vi "Initialize.vi"(8 "error in (no error)":errorcluster, 9 "Variable Names":string[](array[string]), 10 "Description":string, 11 "Pipe Name":string) -> (0 "error out":errorcluster, 3 "Pipe":T1)   [LabVIEW 2022 SP3, in "Pipes.lvlib"]
uses:
  Pipes.lvlib
  Controls/Pipe.ctl
  Controls/Pipe Definition.ctl
  Controls/Token Type.ctl
  Controls/Token.ctl
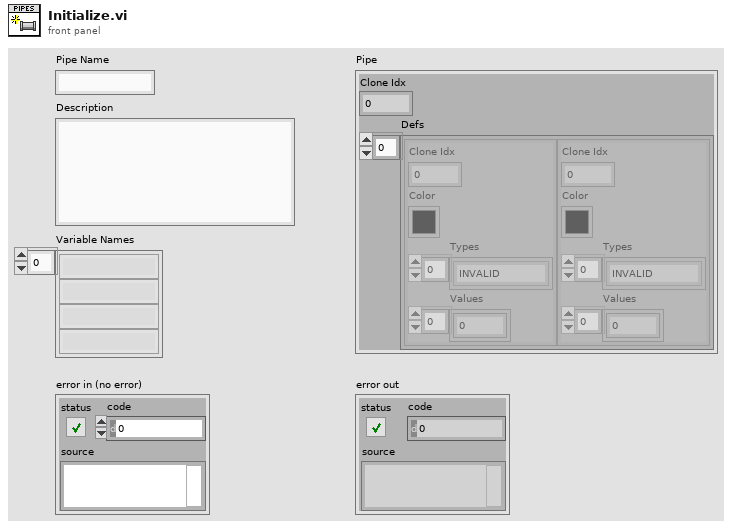
[diagram p1: front panel]
types:
  T1 = typedef "Pipes.lvlib/Pipe.ctl" = cluster{"Clone Idx":i32, "Defs":T2[]}
  T2 = typedef "Pipes.lvlib/Pipe Definition.ctl" = cluster{"Clone Idx":i32, "Color":u32, "Types":T3[], "Values":dbl[]}
  T3 = typedef "Pipes.lvlib/Token Type.ctl" = enum8{"INVALID", "NOT", "AND", "OR", "EE", "NE", "LT", "GT", "LTE", "GTE", "PLUS", "MINUS", "MULTIPLY", "DIVIDE", "MODULUS", "LPAREN", "RPAREN", "LITERAL", "IDENTIFIER", "DEFINITION"}
  T4 = typedef "Pipes.lvlib/Token.ctl" = cluster{"Offset":i32, "Type":T3, "Value":string}
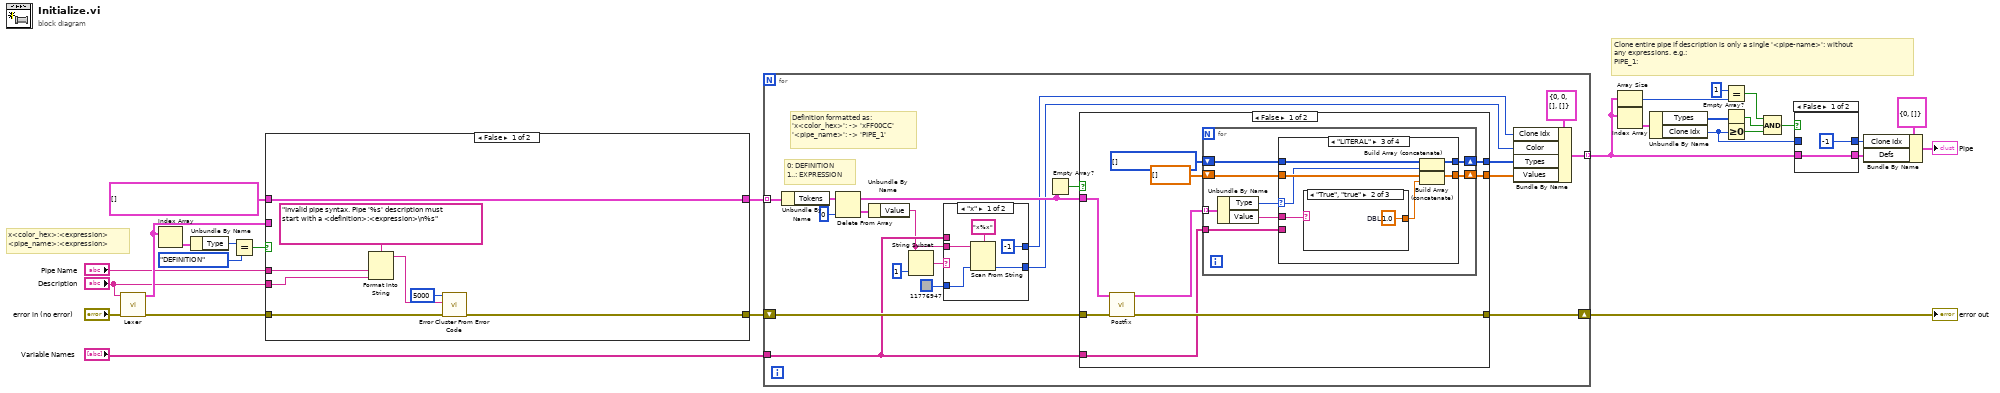
[diagram p0: block diagram]
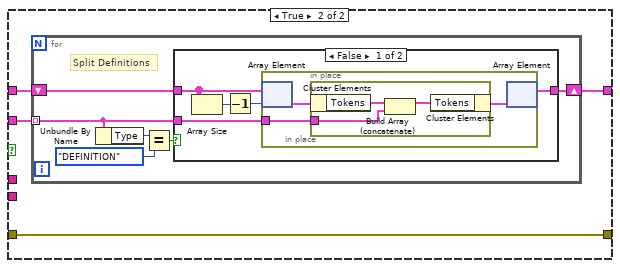
[diagram p3: hidden frame]
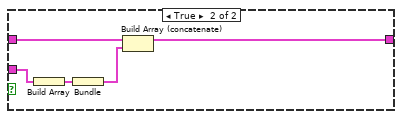
[diagram p4: hidden frame]
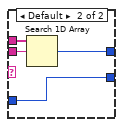
[diagram p5: hidden frame]
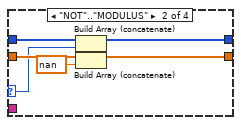
[diagram p7: hidden frame]
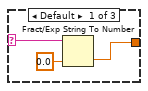
[diagram p8: hidden frame]
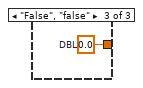
[diagram p9: hidden frame]
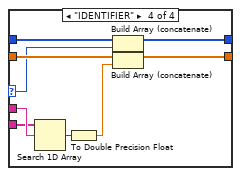
[diagram p10: hidden frame]
diagram:
  # "Clone entire pipe if description is only a single '<pipe-name>': without\nany expressions. e.g.:\nPIPE_1:"
  # "x<color_hex>:<expression>\n<pipe_name>:<expression>"
  n1 = call "Lexer.vi"("error in (no error)"="error in (no error)", "Input"="Description") -> ("error out"=w15:errorcluster, "Tokens"=w21:T4[])  [unwired: 8 in]
  n2 = Index Array(array=w21) -> (element=w18:T4)  [unwired: 1 in]
  n3 = Unbundle By Name(w18) -> ("Type"=w19:T3)
  n4 = Equal?(x=w19, y=Token_Type."DEFINITION" ("x")) -> (x = y?=w17:bool)
  n5 = case shown="False" w17 {
    tunnel: cluster{"Tokens":T4[]}[] [] ("Defs") -> [w35 w40]
    tunnel: [w35 w39] -> w23
    tunnel: w21 -> [_ w38]
    tunnel: [w34 w37] -> w16
    tunnel: w15 -> [w36 w37]
    tunnel: "Description" -> [w30 _]
    tunnel: "Pipe Name" -> [w32 _]
    frame False {
      n6 = Format Into String(format string="Invalid pipe syntax. Pipe '%s' description must start with a <definition>:<expression>\n%s" ("error message (\"\")"), w32, w30) -> (resulting string=w29:string)  [unwired: 2 in, 1 out]
      n7 = call <vilib>:"Error Cluster From Error Code.vi"("error in (no error)"=w36, "error message (\"\")"=w29, "error code (0)"=5000) -> ("error out"=w34:errorcluster)  [unwired: 6 in]
    }
    frame True {
      n8 = for {
        tunnel: w38 -> [w43] mode=indexing
        shift-right: [w42] -> w39
        shift-left: w40 -> [w44]
        # "Split Definitions"
        n9 = Unbundle By Name(w43) -> ("Type"=w46:T3)
        n10 = Equal?(x=w46, y=Token_Type."DEFINITION" ("x")) -> (x = y?=w41:bool)
        n11 = case shown="False" w41 {
          tunnel: w44 -> [w51 w62]
          tunnel: w43 -> [w48 w61]
          tunnel: [w47 w58] -> w42
          frame False {
            n12 = Array Size(array=w51) -> (size(s)=w50:i32)
            n13 = Decrement(x=w50) -> (x-1=w49:i32)
            n14 = in-place {
              in-place-border: w48 -> [w53]
              n15 = in-place-array #1(w51, w49) -> (w54:cluster{"Tokens":T4[]})
              n16 = in-place {
                in-place-border: w53 -> [w55]
                n17 = in-place-cluster #2(w54) -> ("Tokens"=w57:T4[])
                n18 = Build Array (concatenate)(w57, w55) -> (w56:T4[])
                n19 = in-place-cluster #2("Tokens"=w56) -> (w52:cluster{"Tokens":T4[]})
              }
              n20 = in-place-array #1(w52) -> (w47:cluster{"Tokens":T4[]}[])  [unwired: 1 out]
            }
          }
          frame True {
            n21 = Build Array(w61) -> (w60:T4[])
            n22 = Bundle(w60) -> (w59:cluster{T4[]})  [unwired: 1 in]
            n23 = Build Array (concatenate)(w62, w59) -> (w58:cluster{"Tokens":T4[]}[])
          }
        }
      }
    }
  }
  n24 = for {
    shift-right: [w80] -> w25
    shift-left: w16 -> [w81]
    tunnel: w23 -> [w78] mode=indexing
    tunnel: "Variable Names" -> [w69]
    tunnel: [w70] -> w5 mode=indexing
    # "Definition formatted as:\n'x<color_hex>': -> 'xFF00CC'\n'<pipe_name>': -> 'PIPE_1'"
    # "0: DEFINITION\n1..: EXPRESSION"
    n25 = Unbundle By Name(w78) -> ("Tokens"=w77:T4[])
    n26 = Delete From Array(array=w77, index=0) -> (deleted portion=w75:T4, array with subset deleted=w72:T4[])  [unwired: 1 in]
    n27 = Unbundle By Name(w75) -> ("Value"=w68:string)
    n28 = String Subset(string=w68, length (rest)=1 ("length (rest)")) -> (substring=w66:string)  [unwired: 1 in]
    n29 = case shown="\"x\"" w66 {
      tunnel: w69 -> [_ w90]
      tunnel: w68 -> [w86 w89]
      tunnel: [-1 ("index of element") w88] -> w65
      tunnel: [w84 w87] -> w64
      tunnel: u32 11776947 ("Color") -> [w85 w87]
      frame "x" {
        n30 = Scan From String(format string="x%x", input string=w86, default 1=w85) -> (output 1=w84:u32)  [unwired: 2 in, 3 out]
      }
      frame Default {
        n31 = Search 1D Array(1D array=w90, element=w89) -> (index of element=w88:i32)  [unwired: 1 in]
      }
    }
    n32 = Empty Array?(array=w72) -> (empty?=w71:bool)
    n33 = case shown="False" w71 {
      tunnel: w81 -> [w99 w137]
      tunnel: [w98 w137] -> w80
      tunnel: [w95 _] -> w74
      tunnel: [w93 _] -> w73
      tunnel: w69 -> [w92 _]
      tunnel: w72 -> [w91 _]
      frame False {
        w96 = T3[] [] items=["INVALID", "NOT", "AND", "OR", "EE", "NE", "LT", "GT", "LTE", "GTE", "PLUS", "MINUS", "MULTIPLY", "DIVIDE", "MODULUS", "LPAREN", "RPAREN", "LITERAL", "IDENTIFIER", "DEFINITION"]
        n34 = call "Postfix.vi"("error in (no error)"=w99, "Tokens"=w91) -> ("error out"=w98:errorcluster, "Postfix"=w97:T4[])  [unwired: 8 in]
        n35 = for {
          tunnel: w97 -> [w107] mode=indexing
          shift-right: [w105] -> w95
          shift-left: w96 -> [w104]
          shift-right: [w102] -> w93
          shift-left: dbl[] [] ("Values") -> [w103]
          tunnel: w92 -> [w100]
          n36 = Unbundle By Name(w107) -> ("Type"=w106:T3, "Value"=w101:string)
          n37 = case shown="\"LITERAL\"" w106 {
            selector: w106 -> [_ w111 w118 w132]
            tunnel: [w109 w113 w120 w134] -> w105
            tunnel: w104 -> [w109 w115 w122 w136]
            tunnel: w103 -> [w108 w114 w121 w135]
            tunnel: [w108 w112 w119 w133] -> w102
            tunnel: w101 -> [_ _ w117 w131]
            tunnel: w100 -> [_ _ _ w130]
            frame "INVALID", "LPAREN", "RPAREN", "DEFINITION" {
            }
            frame "NOT".."MODULUS" {
              n38 = Build Array (concatenate)(w115, w111) -> (w113:T3[])
              n39 = Build Array (concatenate)(w114, nan) -> (w112:dbl[])
            }
            frame "LITERAL" {
              n40 = case shown="\"True\", \"true\"" w117 {
                selector: w117 -> [w125 _ _]
                tunnel: [w123 w126 w127] -> w116
                frame Default {
                  n41 = Fract/Exp String To Number(string=w125, default (0 dbl)=0.0 ("DBL")) -> (number=w123:dbl)  [unwired: 2 in, 1 out]
                }
                frame "True", "true" {
                  w126 = 1.0  # DBL
                }
                frame "False", "false" {
                  w127 = 0.0  # DBL
                }
              }
              n42 = Build Array (concatenate)(w122, w118) -> (w120:T3[])
              n43 = Build Array (concatenate)(w121, w116) -> (w119:dbl[])
            }
            frame "IDENTIFIER" {
              n44 = Search 1D Array(1D array=w130, element=w131) -> (index of element=w129:i32)  [unwired: 1 in]
              n45 = To Double Precision Float(number=w129) -> (double precision float=w128:dbl)
              n46 = Build Array (concatenate)(w136, w132) -> (w134:T3[])
              n47 = Build Array (concatenate)(w135, w128) -> (w133:dbl[])
            }
          }
        }
      }
      frame True {
      }
    }
    n48 = Bundle By Name(cluster=T2 {"Clone Idx"=0, "Color"=0, "Types"=[], "Values"=[]} ("Definition"), "Clone Idx"=w65, "Color"=w64, "Types"=w74, "Values"=w73) -> (w70:T2)
  }
  "error out" <- w25
  n49 = Array Size(array=w5) -> (size(s)=w11:i32)
  n50 = Index Array(array=w5) -> (element=w12:T2)  [unwired: 1 in]
  n51 = Unbundle By Name(w12) -> ("Types"=w9:T3[], "Clone Idx"=w2:i32)
  n52 = Equal?(x=1 ("y"), y=w11) -> (x = y?=w8:bool)
  n53 = Empty Array?(array=w9) -> (empty?=w1:bool)
  n54 = Greater Or Equal To 0?(x=w2) -> (x >= 0?=w7:bool)
  n55 = Compound Arithmetic op=AND(w8, w1, w7) -> (w4:bool)
  n56 = case shown="False" w4 {
    tunnel: [w138 _] -> w6
    tunnel: w5 -> [w138 _]
    tunnel: w2 -> [_ w140]
    tunnel: [-1 ("Clone Idx") w140] -> w3
    frame False {
    }
    frame True {
    }
  }
  n57 = Bundle By Name(cluster=T1 {"Clone Idx"=0, "Defs"=[]} ("Pipe"), "Clone Idx"=w3, "Defs"=w6) -> (→"Pipe":T1)
